vi "Get SubPanel Reference.vi"(8 "error in (no error)":errorcluster, 11 "Simple Plugin in":refnum<class "Simple Plugin.lvclass">) -> (0 "error out":errorcluster, 2 "VI Ref":refnum<vi>, 3 "Simple Plugin out":refnum<class "Simple Plugin.lvclass">)   [LabVIEW 2011, in "Simple Plugin.lvclass"]
uses:
  Simple Plugin.lvclass
  Generate Signal.vi
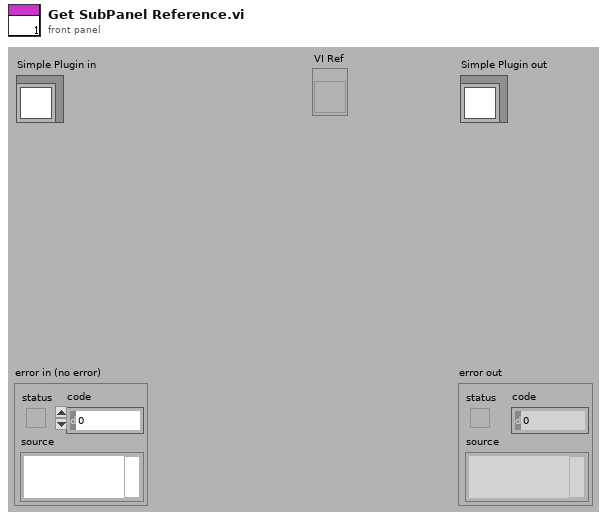
[diagram p1: front panel]
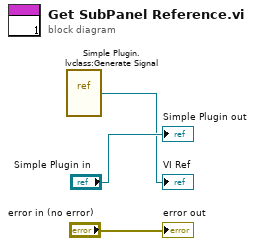
[diagram p0: block diagram]
diagram:
  n1 = vi-ref "Simple Plugin.lvclass:Generate Signal.vi"() -> (→"VI Ref":refnum<vi>)
  "error out" <- "error in (no error)"
  "Simple Plugin out" <- "Simple Plugin in"
